vi "Load Variable Parameters.vi"(11 "Sync Tag In":refnum<class "Synchronised Tag.lvclass">) -> (0 "Error Out":errorcluster, 1 "Node Type":T3, 2 "URL":string, 3 "Sync Tag Out":refnum<class "Synchronised Tag.lvclass">, 4 "SV Data Type":T4, 5 "OPC UA type":T2 items=["Boolean"=1, "SByte"=2, "Byte"=3, "Int16"=4, "UInt16"=5, "Int32"=6, "UInt32"=7, "Int64"=8, "UInt64"=9, "Float"=10, "Double"=11, "String"=12, "DateTime"=13, "ByteString"=15, "Array of Boolean"=101, "Array of SByte"=102, "Array of Byte"=103, "Array of Int16"=104, "Array of UInt16"=105, "Array of Int32"=106, "Array of UInt32"=107, "Array of Int64"=108, "Array of UInt64"=109, "Array of Float"=110, "Array of Double"=111, "Array of String"=112, "Array of DateTime"=113, "Array of ByteString"=115], 6 "Access Mode":T1)   [LabVIEW 2016, in "Synchronised Tag.lvclass"]
uses:
  Synchronised Tag.lvclass
  Controls/SV type.ctl
  Controls/Node Type.ctl
  Controls/OPC type.ctl
  Controls/Access Mode.ctl
  Synchronised Tag.lvclass/Synchronised Tag.ctl
panel:
  in  "error in (no error)":errorcluster
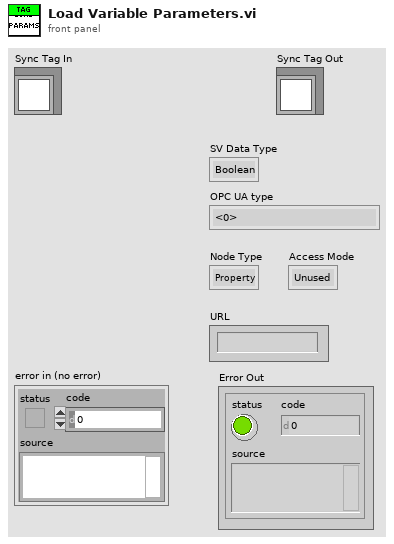
[diagram p1: front panel]
types:
  T1 = typedef "Synchronised Tag.lvclass/Access Mode.ctl" = enum16{"Unused", "Read Only", "Write Only", "Read/Write"}
  T2 = typedef "OPC type.ctl" = u16
  T3 = typedef "Node Type.ctl" = enum16{"Property", "Item", "Folder"}
  T4 = typedef "SV type.ctl" = enum16{"Boolean", "SByte", "Byte", "Int16", "UInt16", "Int32", "UInt32", "Int64", "UInt64", "Float", "Double", "String", "DateTime", "ByteString", "Array of Boolean", "Array of SByte", "Array of Byte", "Array of Int16", "Array of UInt16", "Array of Int32", "Array of UInt32", "Array of Int64", "Array of UInt64", "Array of Float", "Array of Double", "Array of String", "Array of DateTime", "Array of ByteString", "Unsupported"}
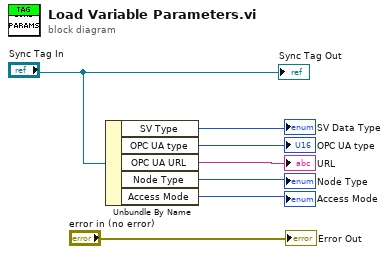
[diagram p0: block diagram]
diagram:
  n1 = Unbundle By Name("Sync Tag In") -> ("SV Type"=→"SV Data Type":T4, "OPC UA type"=→"OPC UA type":T2, "OPC UA URL"=→"URL":string, "Node Type"=→"Node Type":T3, "Access Mode"=→"Access Mode":T1)
  "Error Out" <- "error in (no error)"
  "Sync Tag Out" <- "Sync Tag In"
